vi "tcp_client_UI.vi"(11 "data":refnum<vi>) -> ()   [LabVIEW 2016, in "update.lvlib"]
uses:
  update.lvlib
  tcp_client_data.ctl
  TCP_client/TCP_client.lvclass
  TCP_client/TCP_client.lvclass/TCP_client.ctl
panel:
  out "read":string
  in  "服务器信息":cluster{"host":string, "port":u16}={"host"="121.36.219.111", "port"=10001}
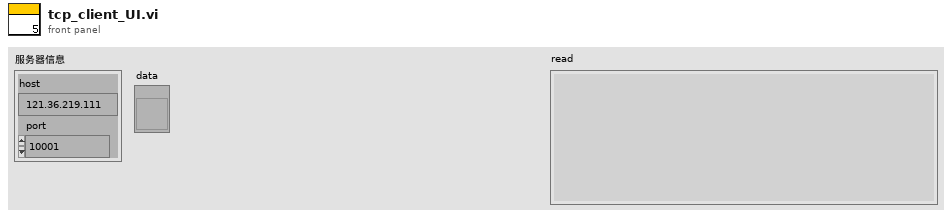
[diagram p1: front panel]
types:
  T1 = typedef "update.lvlib/tcp_client_data.ctl" = cluster{"SPname":string, "MNnumber":string, "Version":string, "state":string}
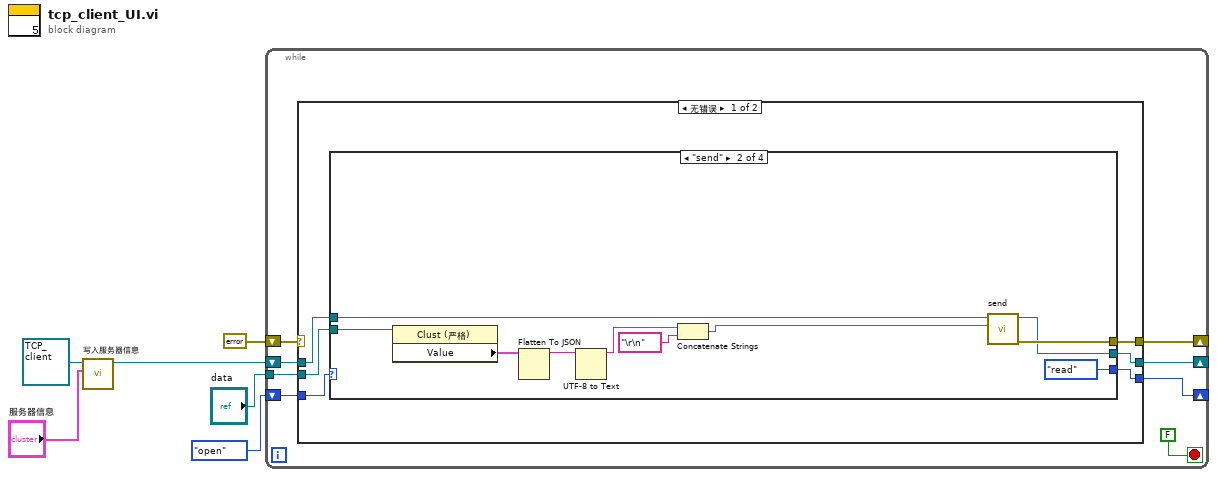
[diagram p0: block diagram]
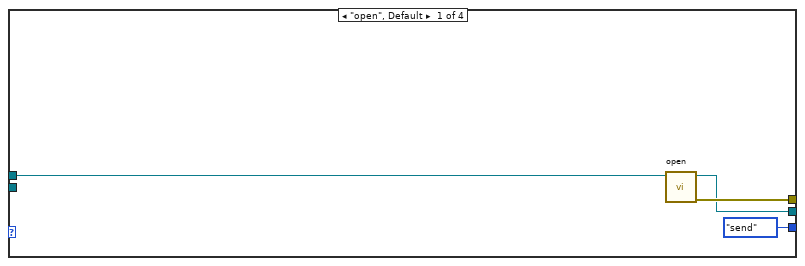
[diagram p2: hidden frame]
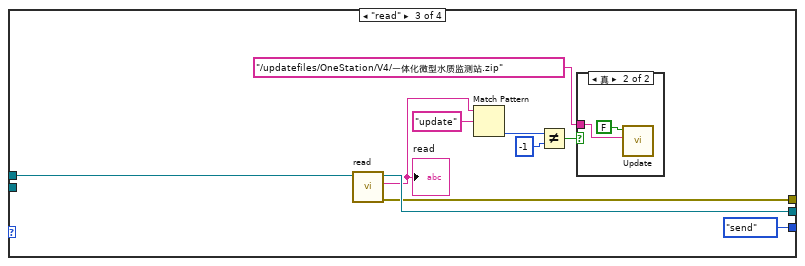
[diagram p3: hidden frame]
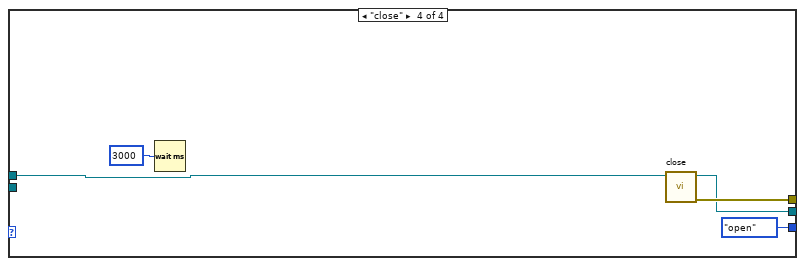
[diagram p5: hidden frame]
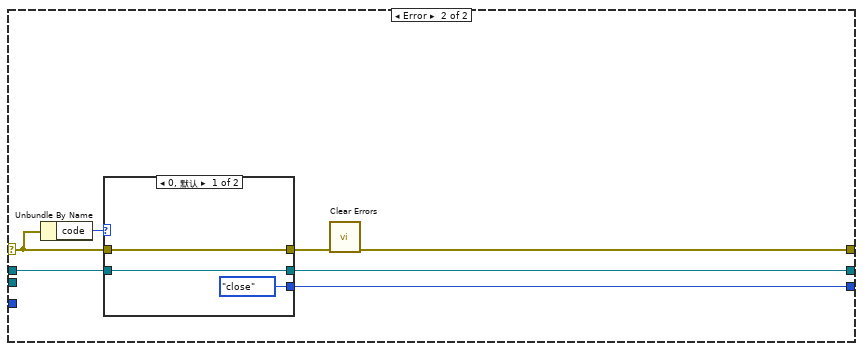
[diagram p6: hidden frame]
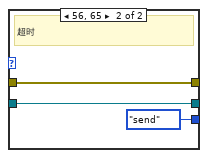
[diagram p7: hidden frame]
diagram:
  n1 = call "写入服务器信息.vi"("服务器信息"="服务器信息", "TCP_client输入"=refnum<class "TCP_client.lvclass"> refnum ("TCP_client.lvclass")) -> ("TCP_client输出"=w4:refnum<class "TCP_client.lvclass">)  [unwired: 8 in, 1 out]
  n2 = while {
    shift-right: [w8] -> _
    shift-left: enum16{"open", "send", "read", "close"}."open" -> [w13]
    shift-right: [w11] -> _
    shift-left: errorcluster {"status"=FALSE, "code"=0, "source"=""} ("error out") -> [w10]
    shift-right: [w9] -> _
    shift-left: w4 -> [w14]
    tunnel: "data" -> [w7]
    stop <- FALSE stop-if-true
    n3 = case shown="无错误" w10 {
      selector: w10 -> [_ w55]
      tunnel: w14 -> [w20 w57]
      tunnel: w13 -> [w19 _]
      tunnel: [w18 w52] -> w11
      tunnel: [w17 w56] -> w9
      tunnel: [w16 w54] -> w8
      tunnel: w7 -> [w15 _]
      frame No Error {
        n4 = case shown="\"send\"" w19 {
          tunnel: w20 -> [w24 w34 w44 w51]
          tunnel: [w23 w33 w42 w50] -> w18
          tunnel: [w22 w32 w43 w49] -> w17
          tunnel: [enum16{"open", "send", "read", "close"}."send" enum16{"open", "send", "read", "close"}."read" enum16{"open", "send", "read", "close"}."send" enum16{"open", "send", "read", "close"}."open"] -> w16
          tunnel: w15 -> [_ w28 _ _]
          frame "open", Default {
            n5 = call-dynamic "open.vi"("TCP_client 输入"=w24) -> ("error out"=w23:errorcluster, "TCP_client 输出"=w22:refnum<class "TCP_client.lvclass">)  [unwired: 9 in]
          }
          frame "send" {
            n6 = property class="Clust (严格)"(reference=w28) -> ("Value"=w25:T1)  [unwired: 1 in, 2 out]
            n7 = Flatten To JSON(anything=w25) -> (JSON string=w27:string)  [unwired: 2 in, 1 out]
            n8 = UTF-8 to Text(11:w27) -> (3:w26:string)  [unwired: 2 in, 1 out]
            n9 = Concatenate Strings(w26, "\r\n" ("字符串")) -> (w29:string)
            n10 = call-dynamic "send.vi"("send"=w29, "TCP_client 输入"=w34) -> ("error out"=w33:errorcluster, "TCP_client 输出"=w32:refnum<class "TCP_client.lvclass">)  [unwired: 8 in]
          }
          frame "read" {
            n11 = call-dynamic "read.vi"("TCP_client 输入"=w44) -> ("error out"=w42:errorcluster, "read"=w40:string, "TCP_client 输出"=w43:refnum<class "TCP_client.lvclass">)  [unwired: 8 in]
            "read" <- w40
            n12 = Match Pattern(string=w40, regular expression="update" ("正则表达式")) -> (offset past match=w38:i32)  [unwired: 1 in, 3 out]
            n13 = Not Equal?(x=w38, y=-1) -> (x != y?=w36:bool)
            n14 = case shown="真" w36 {
              tunnel: "/updatefiles/OneStation/V4/一体化微型水质监测站.zip" ("更新包远端地址") -> [_ w46]
              frame False {
              }
              frame True {
                n15 = call "Update.vi"("更新包远端地址"=w46, "测试版？"=FALSE) -> ()  [unwired: 10 in]
              }
            }
          }
          frame "close" {
            n16 = Wait (ms)(milliseconds to wait=u32 3000 ("等待时间（毫秒）")) -> ()  [unwired: 1 out]
            n17 = call-dynamic "close.vi"("TCP_client 输入"=w51) -> ("error out"=w50:errorcluster, "TCP_client 输出"=w49:refnum<class "TCP_client.lvclass">)  [unwired: 9 in]
          }
        }
      }
      frame Error {
        n18 = Unbundle By Name(w55) -> ("code"=w58:i32)
        n19 = case shown="0, 默认" w58 {
          tunnel: w57 -> [w60 w64]
          tunnel: [w60 w64] -> w56
          tunnel: [w59 w62] -> w53
          tunnel: w55 -> [w59 w62]
          tunnel: [enum16{"open", "send", "read", "close"}."close" enum16{"open", "send", "read", "close"}."send"] -> w54
          frame 0, Default {
          }
          frame 56, 65 {
            # "超时"
          }
        }
        n20 = call <vilib>:"Clear Errors.vi"("error in (no error)"=w53) -> ("error out"=w52:errorcluster)  [unwired: 5 in, 1 out]
      }
    }
  }
